vi "Update.vi"(8 "error in (no error)":errorcluster, 10 "Engine in":refnum<class "Engine.lvclass">, 11 "PongDemo in":refnum<class "PongDemo.lvclass">) -> (0 "error out":errorcluster, 2 "Engine out":refnum<class "Engine.lvclass">, 3 "PongDemo out":refnum<class "PongDemo.lvclass">)   [LabVIEW 2019, in "RT_Game.lvlib" / "PongDemo.lvclass"]
uses:
  PongDemo.lvclass
  C:/Users/FreshBob/Dropbox/VIs/myRIO_GameConsole/RT/RT_Game/Game/Game.lvclass
  Engine/Engine.lvclass
  Game/Game.lvclass/Game.ctl
  AttractScreen/AttractScreen.lvclass
  Engine/Engine.lvclass/Engine.ctl
  Engine/Write NextGame.vi
  Engine/Write SwitchGame_.vi
  Game/Read State.vi
  Pong/Pong.lvclass
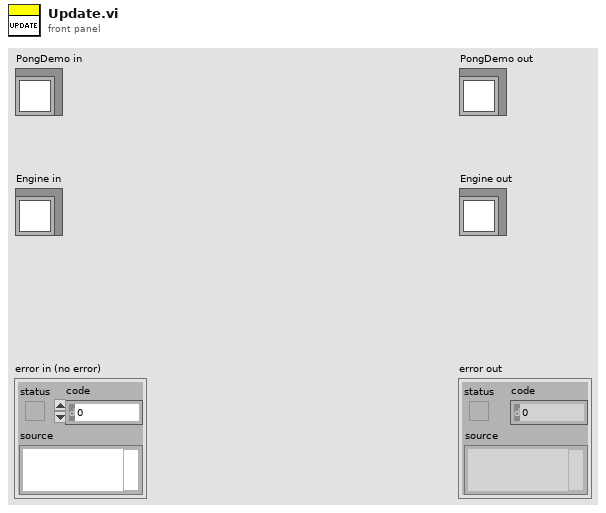
[diagram p1: front panel]
types:
  T1 = typedef "RT_Game.lvlib/Game.lvclass/States.ctl" = enum16{"Init", "Restart", "Menu", "Game", "Resume", "ToggleSingleplayer", "LoadNextGame", "ExitToMenu", "NewHighscore", "GameOver", "SlideOut", "FadeToMenu", "StartFadeToMenu"}
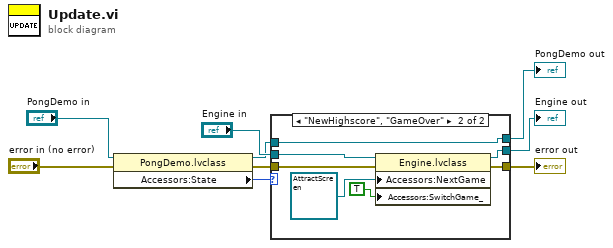
[diagram p0: block diagram]
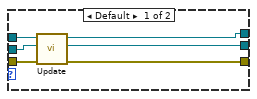
[diagram p2: hidden frame]
diagram:
  n1 = property class="PongDemo.lvclass"(reference="PongDemo in", error in="error in (no error)") -> (reference out=w2:refnum<class "PongDemo.lvclass">, error out=w5:errorcluster, "Accessors:State"=w6:T1)
  n2 = case shown="\"NewHighscore\", \"GameOver\"" w6 {
    tunnel: w5 -> [w15 w22]
    tunnel: [w14 w21] -> w4
    tunnel: "Engine in" -> [w11 w20]
    tunnel: [w10 w19] -> w3
    tunnel: w2 -> [w13 w16]
    tunnel: [w12 w16] -> w1
    frame Default {
      n3 = call-parent "Update.vi"("error in (no error)"=w15, "Engine in"=w11, "Pong in"=w13) -> ("error out"=w14:errorcluster, "Engine out"=w10:refnum<class "Engine.lvclass">, "Pong out"=w12:refnum<class "PongDemo.lvclass">)  [unwired: 6 in]
    }
    frame "NewHighscore", "GameOver" {
      n4 = property class="Engine.lvclass"(reference=w20, error in=w22, "Accessors:NextGame"=refnum<class "AttractScreen.lvclass"> refnum ("RT_Game.lvlib:AttractScreen.lvclass"), "Accessors:SwitchGame_"=TRUE ("SwitchGame_")) -> (reference out=w19:refnum<class "Engine.lvclass">, error out=w21:errorcluster)
    }
  }
  "error out" <- w4
  "PongDemo out" <- w1
  "Engine out" <- w3
